vi "DSF.Engine.Framework.Get Cache.vi"(11 "Framework in":refnum<class "DSF.Engine.Framework.lvclass">) -> (2 "Cache":refnum<class "Memory Cache.lvclass">, 3 "Framework out":refnum<class "DSF.Engine.Framework.lvclass">)   [LabVIEW 2017, in "Data Sharing Framework Engine.lvlib" / "DSF.Engine.Framework.lvclass"]
uses:
  DSF.Engine.Framework.lvclass
  Source/Data Sharing Framework Core/Engine/Memory/Memory Cache/Memory Cache.lvclass
  DSF.Engine.Framework.lvclass/DSF.Engine.Framework.ctl
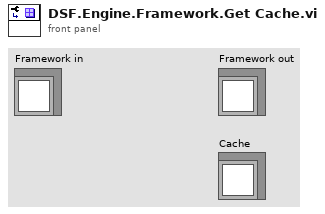
[diagram p1: front panel]
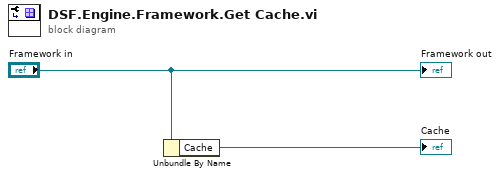
[diagram p0: block diagram]
diagram:
  n1 = Unbundle By Name("Framework in") -> ("Cache"=→"Cache":refnum<class "Memory Cache.lvclass">)
  "Framework out" <- "Framework in"
